vi "SVM_SWLDA_통합버전.vi"(7 "WEIGHT":dbl[](array[numeric]), 8 "svm_parameter":T1={"svm_type"=0, "kernel_type"=3, "degree"=3, "gamma"=0.07, "coef0"=0.0, "cache_size"=100.0, "epsilon"=0.001, "C"=1.0, "nr_weight"=0, "weight_label"=[1, 12], "Weight (C(class i))"=[1.0, 1.0], "nu"=0.5, "p"=0.1, "Shrinking"=1, "probability"=1} {"p" format="%.4f"; "nu" format="%.4f"; "Weight (C(class i))" format="%.2f"; "C" format="%.2f"; "epsilon" format="%.4f"; "cache_size" format="%.2f"; "coef0" format="%.2f"; "gamma" format="%.5f"; "kernel_type" items=["Linear", "Poly", "RBF", "Sigmoid"]; "svm_type" items=["C-SVC", "Nu-SVC", "One-class SVM", "epsilon-SVR", "nu-SVR"]}, 9 "ModelFileName":string="C:\\\\WORK\\\\RBFModel", 10 "ERP_Parameters_of_Target":dbl[][](array[numeric]) format="%0.3f", 11 "ERP_Parameters_of_Nontarget":dbl[][](array[numeric]) format="%0.3f") -> ()   [LabVIEW 2014]
panel:
  out "Array":dbl[][](array[numeric])
  out "Length":i32=12
  # "Results"
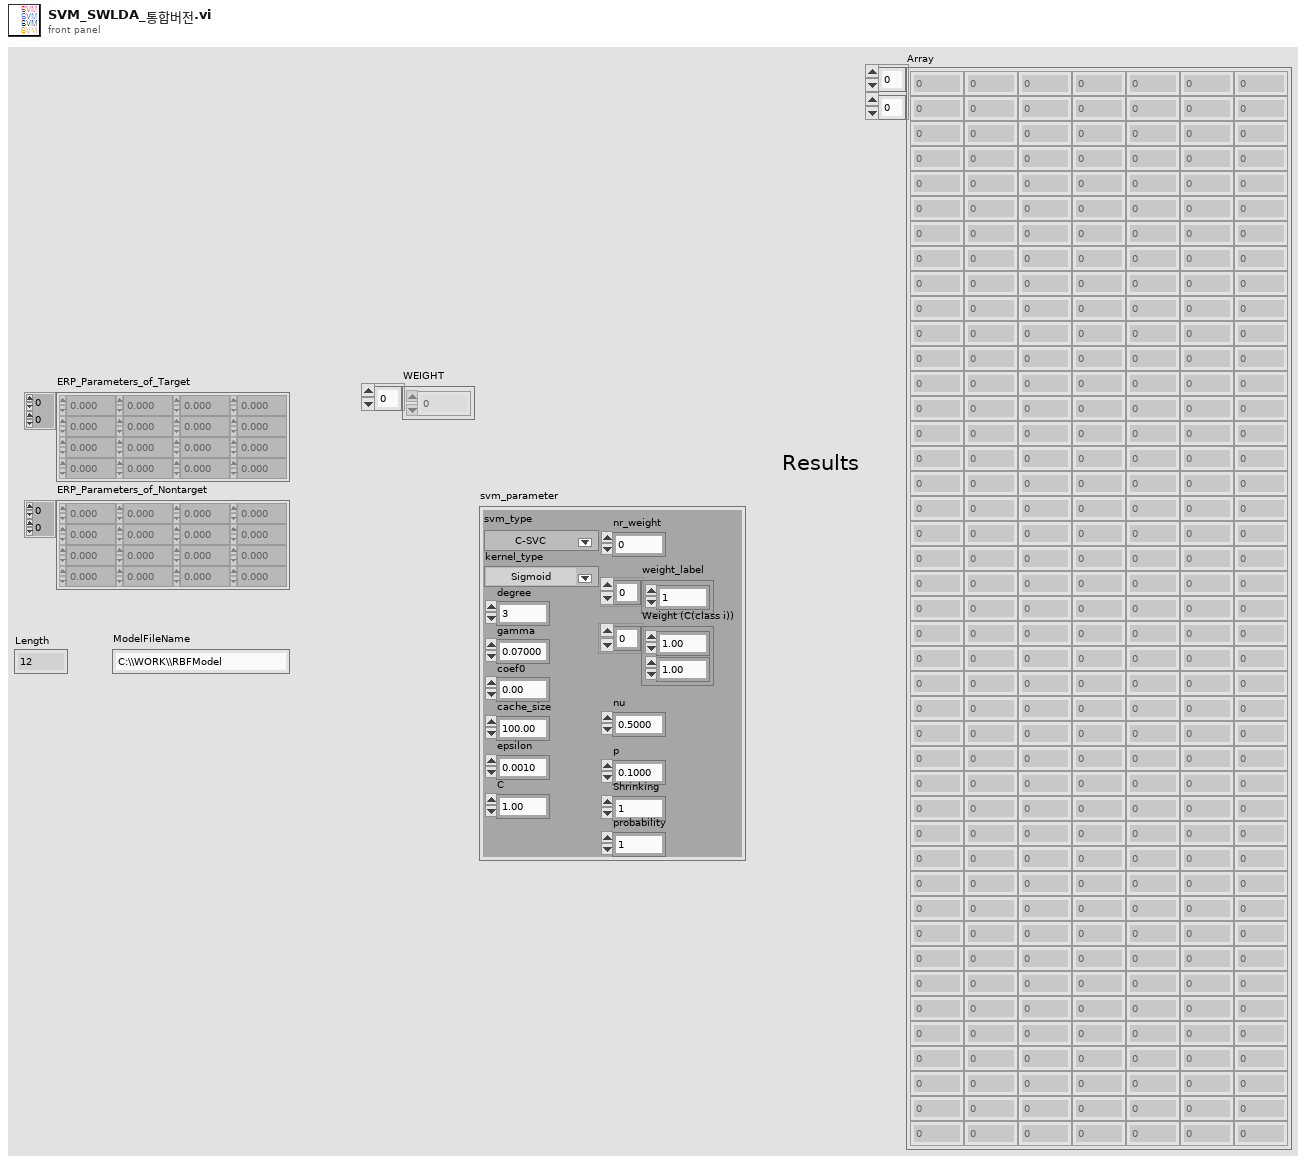
[diagram p1: front panel]
types:
  T1 = cluster{"svm_type":i16, "kernel_type":i16, "degree":i16, "gamma":dbl, "coef0":dbl, "cache_size":dbl, "epsilon":dbl, "C":dbl, "nr_weight":i16, "weight_label":i16[], "Weight (C(class i))":dbl[], "nu":dbl, "p":dbl, "Shrinking":i16, "probability":i16}
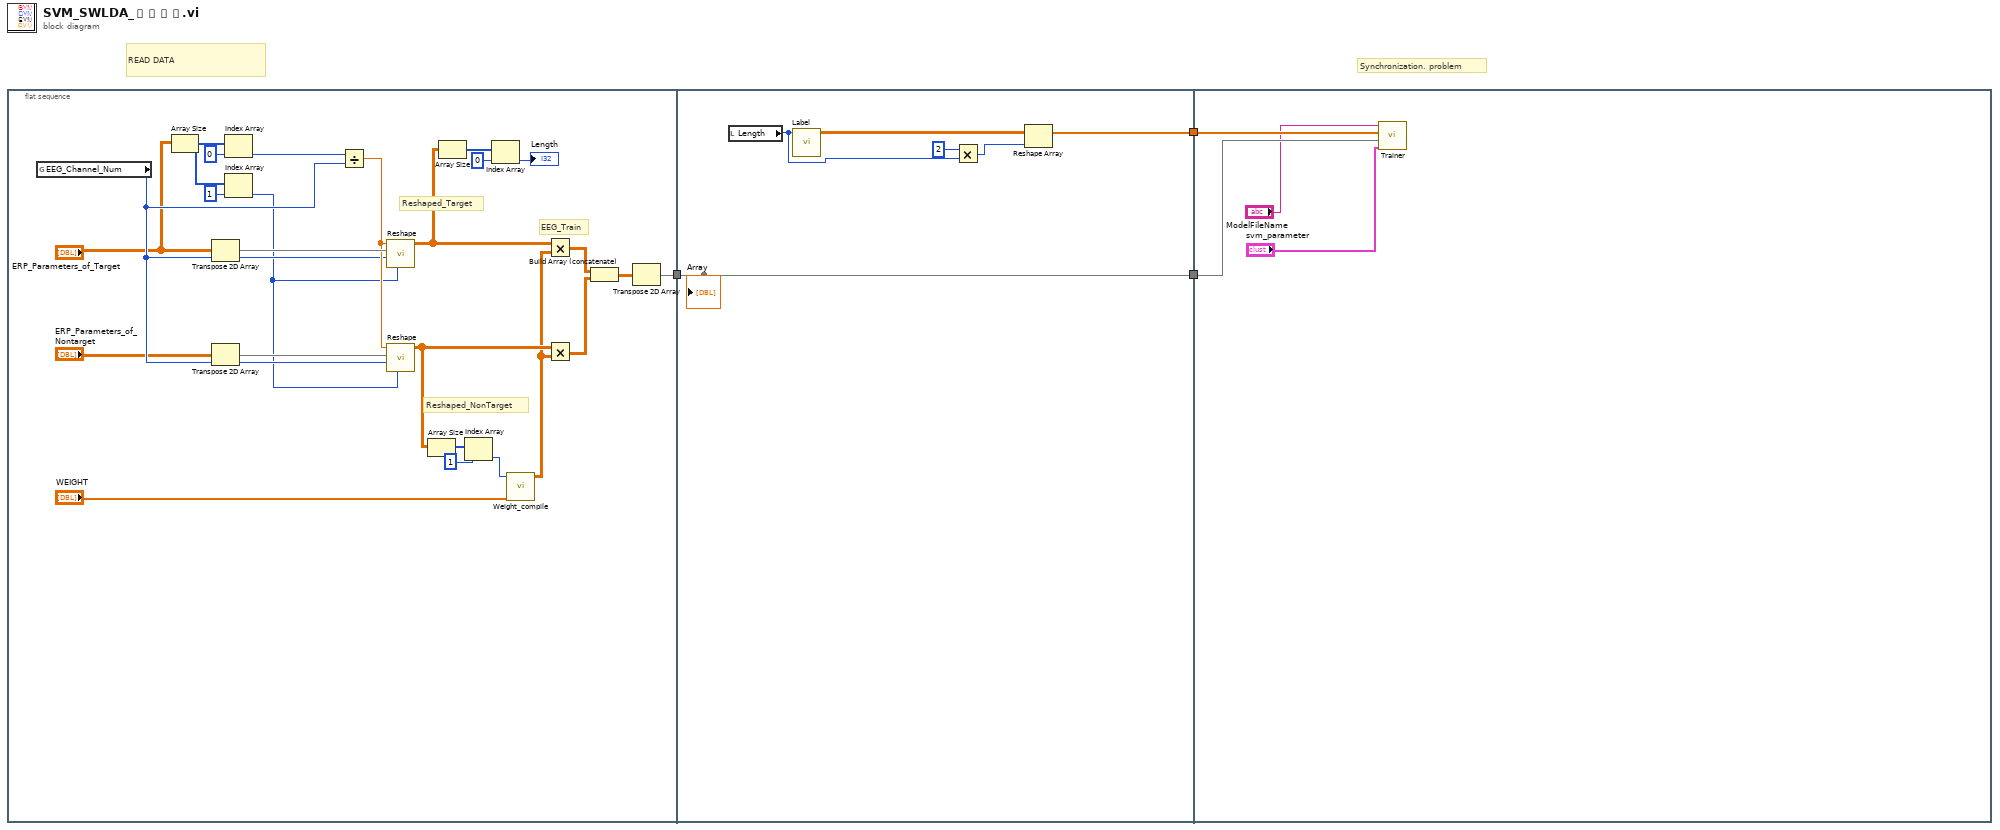
[diagram p0: block diagram]
diagram:
  # "Synchronization. problem"
  # "READ DATA"
  n1 = flat-sequence {
    tunnel: [w19] -> w3
    tunnel: w3 -> [w34]
    tunnel: [w34] -> w2
    tunnel: [w32] -> w1
    tunnel: w2 -> [w37]
    tunnel: w1 -> [w38]
    frame #0 {
      # "EEG_Train"
      # "Reshaped_NonTarget"
      # "Reshaped_Target"
      n2 = global read "Control_Panel.vi" "EEG_Channel_Num"() -> (w17:i32)
      n3 = Array Size(array="ERP_Parameters_of_Target") -> (size(s)=w26:i32[])
      n4 = Transpose 2D Array(2D array="ERP_Parameters_of_Target") -> (transposed array=w22:dbl[][])
      n5 = Transpose 2D Array(2D array="ERP_Parameters_of_Nontarget") -> (transposed array=w21:dbl[][])
      n6 = Index Array(array=w26, index=0) -> (element=w25:i32)
      n7 = Index Array(array=w26, index=1) -> (element=w16:i32)
      n8 = Divide(x=w25, y=w17) -> (x/y=w18:dbl)
      n9 = call "Reshape.vi"("Numeric"=w16, "EEG_Channel_Num"=w17, "all rows"=w22, "Numeric 2"=w18) -> ("Array"=w6:dbl[][])  [unwired: 7 in]
      n10 = call "Reshape.vi"("Numeric"=w16, "EEG_Channel_Num"=w17, "all rows"=w21, "Numeric 2"=w18) -> ("Array"=w11:dbl[][])  [unwired: 7 in]
      n11 = Array Size(array=w11) -> (size(s)=w10:i32[])
      n12 = Array Size(array=w6) -> (size(s)=w23:i32[])
      n13 = Index Array(array=w10, index=1) -> (element=w8:i32)
      n14 = Index Array(array=w23, index=0) -> (element=→"Length":i32)
      n15 = call "Weight_compile.vi"("WEIGHT"="WEIGHT", "column_number"=w8) -> ("Compiled_weight"=w4:dbl[][])  [unwired: 9 in]
      n16 = Multiply(x=w6, y=w4) -> (x*y=w5:dbl[][])
      n17 = Multiply(x=w11, y=w4) -> (x*y=w7:dbl[][])
      n18 = Build Array (concatenate)(w5, w7) -> (w15:dbl[][])
      n19 = Transpose 2D Array(2D array=w15) -> (transposed array=w19:dbl[][])
    }
    frame #1 {
      n20 = local read "Length"() -> (w30:i32)
      n21 = call "Label.vi"("Numeric"=w30) -> ("Array"=w33:dbl[][])  [unwired: 10 in]
      n22 = Multiply(x=2, y=w30) -> (x*y=w31:i32)
      n23 = Reshape Array(w33, w31) -> (w32:dbl[])
      "Array" <- w34
    }
    frame #2 {
      n24 = call "Trainer.vi"("svm_parameter"="svm_parameter", "attributes"=w37, "Lables"=w38, "ModelFileName"="ModelFileName") -> ()
    }
  }
